vi "RenameBook.vi"(2 "Parameters":T1={"Book Folder Name"="", "Full file name"="", "Remote Path"="bookfiles/", "Shelf folder"=path "", "Existing books"=[], "Dialog?"=enum."No Dialog", "New Format?"=FALSE}, 3 "base path":path, 4 "error in":errorcluster) -> (0 "error out":errorcluster, 1 "destination":path)   [LabVIEW 2012]
uses:
  <userlib>/BotSpeak/Devices/EvalRIO/FTPCodes/FTPParameters.ctl
panel:
  out "target":path
  out "source":path
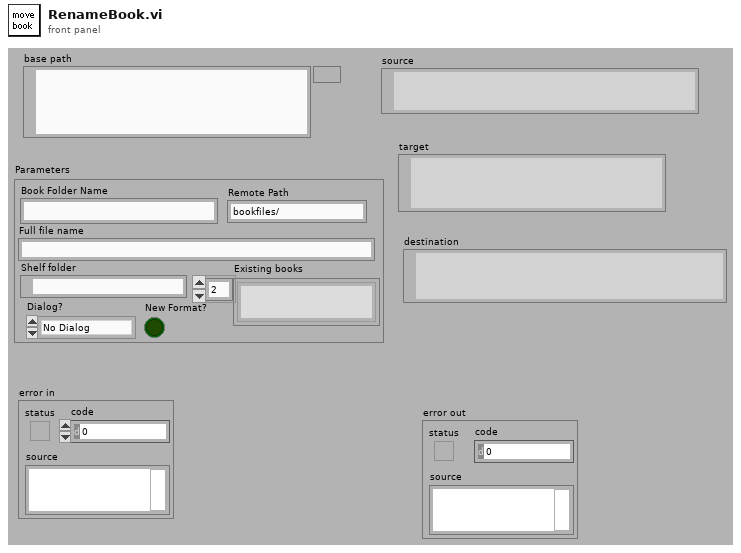
[diagram p1: front panel]
types:
  T1 = typedef "FTPParameters.ctl" = cluster{"Book Folder Name":string, "Full file name":string, "Remote Path":string, "Shelf folder":path, "Existing books":string[], "Dialog?":enum16{"No Dialog", "Dialog", "Overwrite"}, "New Format?":bool}
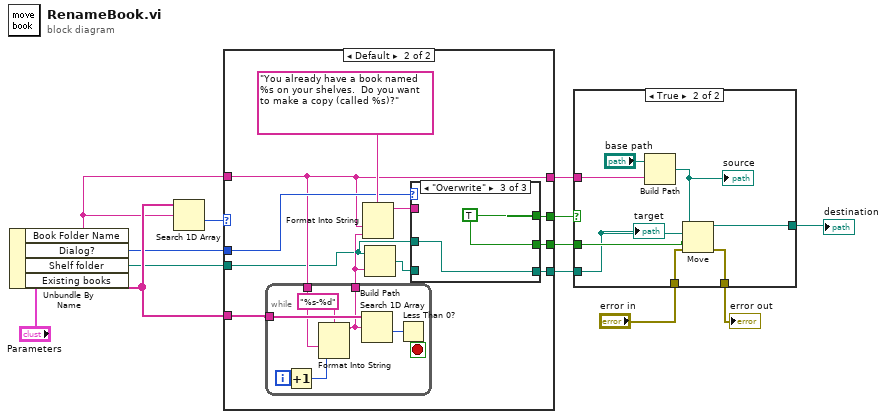
[diagram p0: block diagram]
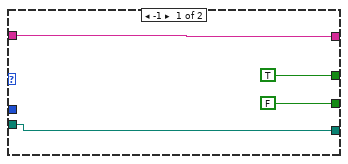
[diagram p2: hidden frame]
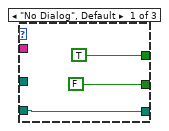
[diagram p3: hidden frame]
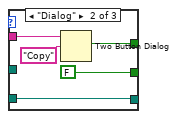
[diagram p4: hidden frame]
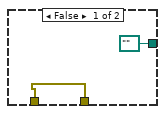
[diagram p5: hidden frame]
diagram:
  n1 = Unbundle By Name("Parameters") -> ("Book Folder Name"=w4:string, "Dialog?"=w5:enum16{"No Dialog", "Dialog", "Overwrite"}, "Shelf folder"=w2:path, "Existing books"=w6:string[])
  n2 = Search 1D Array(1D array=w6, element=w4) -> (index of element=w9:i32)  [unwired: 1 out]
  n3 = case shown="Default" w9 {
    tunnel: [TRUE ("T button?") w26] -> w11
    tunnel: w6 -> [_ w25]
    tunnel: w4 -> [w16 w22]
    tunnel: [w16 w22] -> w8
    tunnel: w5 -> [_ w24]
    tunnel: [FALSE ("T button?") w23] -> w3
    tunnel: w2 -> [w14 w18]
    tunnel: [w14 w19] -> w1
    frame -1 {
    }
    frame Default {
      n4 = while {
        tunnel: w25 -> [w45]
        tunnel: [w40] -> w21
        tunnel: w22 -> [w39]
        i -> [w42]
        stop <- w44 stop-if-true
        n5 = Increment(x=w42) -> (x+1=w41:i32)
        n6 = Format Into String(format string="%s-%d", w39, w41) -> (resulting string=w40:string)  [unwired: 2 in, 1 out]
        n7 = Search 1D Array(1D array=w45, element=w40) -> (index of element=w46:i32)  [unwired: 1 out]
        n8 = Less Than 0?(x=w46) -> (x < 0?=w44:bool)
      }
      n9 = Format Into String(format string="You already have a book named %s on your shelves.  Do you want to make a copy (called %s)?", w22, w21) -> (resulting string=w28:string)  [unwired: 2 in, 1 out]
      n10 = Build Path(base path=w18, name or relative path=w21) -> (appended path=w20:path)
      n11 = case shown="\"Overwrite\"" w24 {
        tunnel: w28 -> [_ w35 _]
        tunnel: [TRUE ("T button?") w34 w38] -> w26
        tunnel: [FALSE ("T button?") FALSE ("T button?") w38] -> w23
        tunnel: [w29 w32 w37] -> w19
        tunnel: w20 -> [w29 w32 _]
        tunnel: w18 -> [_ _ w37]
        frame "No Dialog", Default {
        }
        frame "Dialog" {
          n12 = Two Button Dialog(message=w35, 2:"Copy" ("T button name (\"OK\")")) -> (T button?=w34:bool)  [unwired: 1 out]
        }
        frame "Overwrite" {
          w38 = TRUE ("T button?")
        }
      }
    }
  }
  n13 = case shown="True" w11 {
    tunnel: [w48 w56] -> w13
    tunnel: "error in" -> [w48 w55]
    tunnel: w8 -> [_ w54]
    tunnel: [path "" ("new path") w53] -> w10
    tunnel: w3 -> [_ w50]
    tunnel: w1 -> [_ w49]
    frame False {
    }
    frame True {
      n14 = Build Path(base path="base path", name or relative path=w54) -> (appended path=w51:path)
      "source" <- w51
      n15 = Move(source path=w51, error in=w55, 9:w50, 10:w49) -> (error out=w56:errorcluster, 3:w53:path)  [unwired: 2 out]
      "target" <- w49
    }
  }
  "error out" <- w13
  "destination" <- w10
